vi "FTW-Endpoint-IncomingRequestProxy-Worker.vi"(1 "Backend":refnum<user-event>, 2 "Frontend Endpoint":refnum<class "FTW-Endpoint.lvclass">) -> ()   [LabVIEW 2013, in "FTW-Actor.lvlib" / "FTW-Endpoint.lvclass"]
uses:
  FTW-Endpoint.lvclass
  Message/Request/FTW-Message-IncomingRequest.lvclass
panel:
  out "Iteration":i32
  out "Messages Handled":i32
  # "Inputs"
  # "Debug"
  # "Outputs"
  # "This asynchronous worker has no outputs"
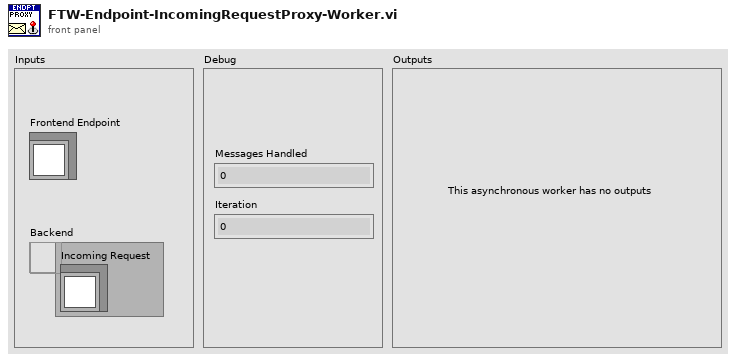
[diagram p1: front panel]
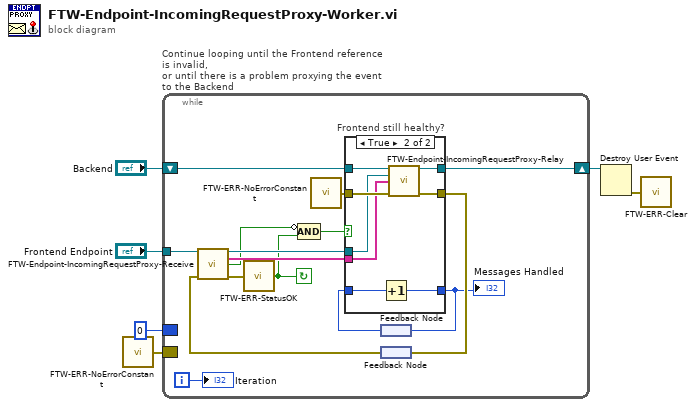
[diagram p0: block diagram]
diagram:
  n1 = call "FTW-ERR-NoErrorConstant.vi"() -> ("no error"=w4:errorcluster)
  n2 = while "Continue looping until the Frontend reference is invalid,\nor until there is a problem proxying the event to the Backend" {
    tunnel: "Frontend Endpoint" -> [w20]
    border: w4 -> [_]
    shift-right: [w15] -> w3
    shift-left: "Backend" -> [w21]
    border: 0 ("Messages Handled") -> [_]
    i -> [w8]
    stop <- w11 continue-if-true
    n3 = call "FTW-ERR-NoErrorConstant.vi"() -> ("no error"=w14:errorcluster)
    n4 = feedback #1() -> (w7:i32)
    n5 = feedback #2() -> (w18:errorcluster)
    n6 = call-dynamic "FTW-Endpoint-IncomingRequestProxy-Receive.vi"("FTW Endpoint"=w20, "error in"=w18) -> ("FTW Endpoint out"=w13:refnum<class "FTW-Endpoint.lvclass">, "Message Received"=w16:string[], "Timed out?"=w12:bool, "error out"=w19:errorcluster)  [unwired: 10 in]
    n7 = call "FTW-ERR-StatusOK.vi"("error to check"=w19) -> ("Status OK?"=w11:bool)
    n8 = Compound Arithmetic op=AND(invert w12, w11) -> (w10:bool)
    n9 = case "Frontend still healthy?" shown="True" w10 {
      tunnel: w21 -> [w24 w32]
      tunnel: [w23 w29] -> w17
      tunnel: w16 -> [_ w28]
      tunnel: [w24 w31] -> w15
      tunnel: w14 -> [w23 w30]
      tunnel: w13 -> [_ w27]
      tunnel: [w22 w26] -> w9
      tunnel: w7 -> [w22 w25]
      frame False {
      }
      frame True {
        n10 = Increment(x=w25) -> (x+1=w26:i32)
        n11 = call "FTW-Endpoint-IncomingRequestProxy-Relay.vi"("Incoming Request Event"=w32, "Frontend Endpoint"=w27, "Multipart Message"=w28, "error in"=w30) -> ("Incoming Request Event out"=w31:refnum<user-event>, "error out"=w29:errorcluster)  [unwired: 10 in]
      }
    }
    "Messages Handled" <- w9
    n12 = feedback-in #1(w9) -> ()
    n13 = feedback-in #2(w17) -> ()
    "Iteration" <- w8
  }
  n14 = Destroy User Event(user event=w3) -> (error out=w2:errorcluster)  [unwired: 1 in]
  n15 = call "FTW-ERR-Clear.vi"("error to snuff"=w2) -> ()  [unwired: 1 out]
